vi "OA Set Int.vi"(8 "error in (no error)":errorcluster, 9 "iIntValue":i32, 10 "pcModeParam":string, 11 "pcModeName":string) -> (0 "error out":errorcluster, 3 "function return":u32)   [LabVIEW 2014, in "atmcd32d.lvlib"]
doc: "unsigned int WINAPI OA_SetInt(const char * const pcModeName, const char * pcModeParam, const int iIntValue);"
uses:
  atmcd32d.lvlib
  atmcd32d.dll
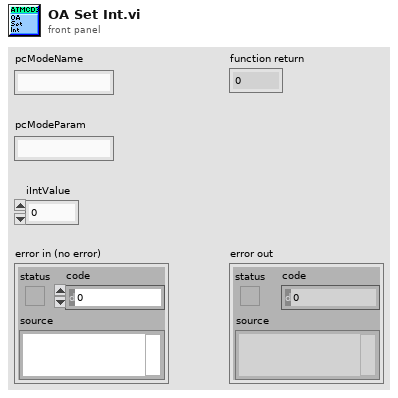
[diagram p1: front panel]
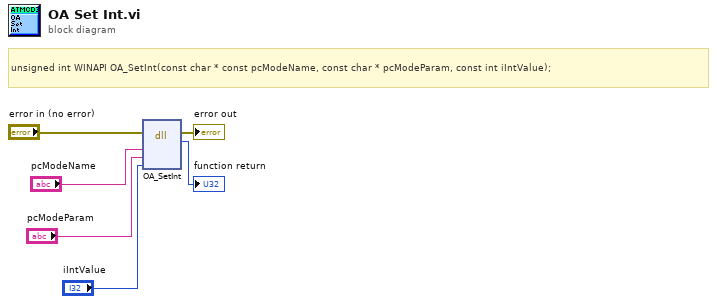
[diagram p0: block diagram]
diagram:
  # "unsigned int WINAPI OA_SetInt(const char * const pcModeName, const char * pcModeParam, const int iIntValue);"
  n1 = dll-call lib="C:/Users/Bakir/Documents/Lambda2-Testing/lib/Andorlib/atmcd32d.*" fn="OA_SetInt"(error in="error in (no error)", "pcModeName"="pcModeName", "pcModeParam"="pcModeParam", "iIntValue"="iIntValue") -> (error out=→"error out":errorcluster, →"function return":u32)  [unwired: 5 in, 1 out]
